vi "Read Inputs from system.vi"(8 "error in":errorcluster, 11 "GPIC Core runtime in":refnum<class "GPIC Core runtime.lvclass">) -> (0 "error out":errorcluster, 2 "Inputs from system":T1, 3 "GPIC Core runtime out":refnum<class "GPIC Core runtime.lvclass">)   [LabVIEW 2017, in "GPIC Core runtime.lvclass"]
uses:
  GPIC Core runtime.lvclass
  configuration/input data indices.ctl
  GPIC Core runtime.lvclass/GPIC Core runtime.ctl
  configuration/GPIC Core configuration.lvclass
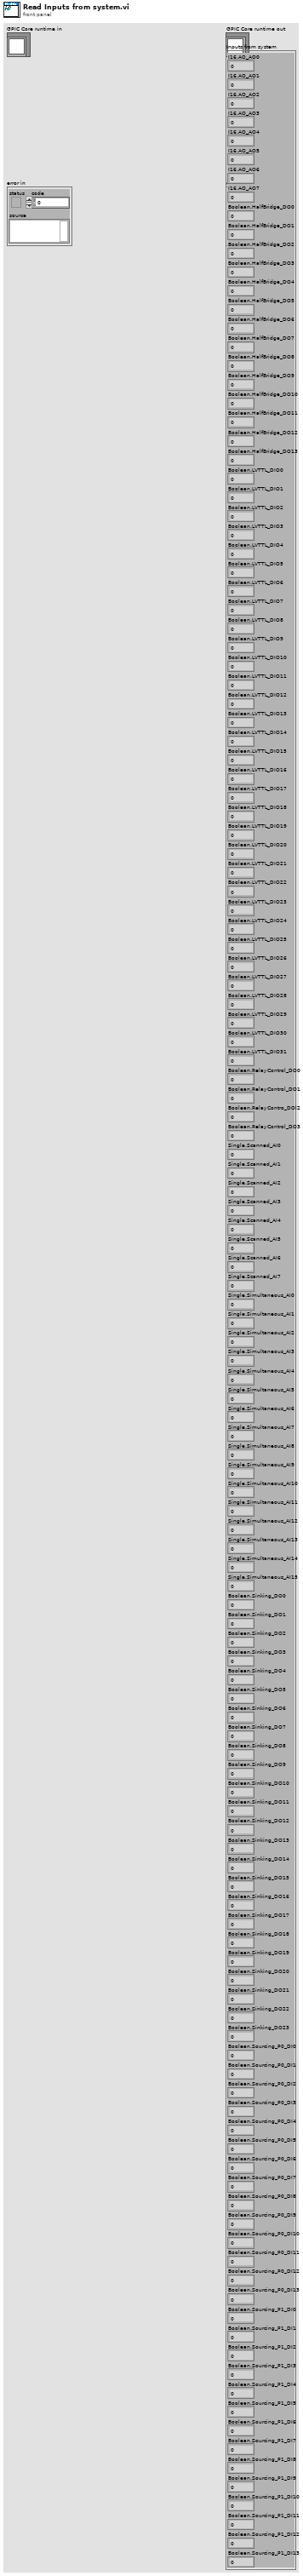
[diagram p1: front panel]
types:
  T1 = typedef "GPIC Core configuration.lvclass/input data indices.ctl" = cluster{"I16.AO_AO0":i32, "I16.AO_AO1":i32, "I16.AO_AO2":i32, "I16.AO_AO3":i32, "I16.AO_AO4":i32, "I16.AO_AO5":i32, "I16.AO_AO6":i32, "I16.AO_AO7":i32, "Boolean.HalfBridge_DO0":i32, "Boolean.HalfBridge_DO1":i32, "Boolean.HalfBridge_DO2":i32, "Boolean.HalfBridge_DO3":i32, "Boolean.HalfBridge_DO4":i32, "Boolean.HalfBridge_DO5":i32, "Boolean.HalfBridge_DO6":i32, "Boolean.HalfBridge_DO7":i32, "Boolean.HalfBridge_DO8":i32, "Boolean.HalfBridge_DO9":i32, "Boolean.HalfBridge_DO10":i32, "Boolean.HalfBridge_DO11":i32, "Boolean.HalfBridge_DO12":i32, "Boolean.HalfBridge_DO13":i32, "Boolean.LVTTL_DIO0":i32, "Boolean.LVTTL_DIO1":i32, "Boolean.LVTTL_DIO2":i32, "Boolean.LVTTL_DIO3":i32, "Boolean.LVTTL_DIO4":i32, "Boolean.LVTTL_DIO5":i32, "Boolean.LVTTL_DIO6":i32, "Boolean.LVTTL_DIO7":i32, "Boolean.LVTTL_DIO8":i32, "Boolean.LVTTL_DIO9":i32, "Boolean.LVTTL_DIO10":i32, "Boolean.LVTTL_DIO11":i32, "Boolean.LVTTL_DIO12":i32, "Boolean.LVTTL_DIO13":i32, "Boolean.LVTTL_DIO14":i32, "Boolean.LVTTL_DIO15":i32, "Boolean.LVTTL_DIO16":i32, "Boolean.LVTTL_DIO17":i32, "Boolean.LVTTL_DIO18":i32, "Boolean.LVTTL_DIO19":i32, "Boolean.LVTTL_DIO20":i32, "Boolean.LVTTL_DIO21":i32, "Boolean.LVTTL_DIO22":i32, "Boolean.LVTTL_DIO23":i32, "Boolean.LVTTL_DIO24":i32, "Boolean.LVTTL_DIO25":i32, "Boolean.LVTTL_DIO26":i32, "Boolean.LVTTL_DIO27":i32, "Boolean.LVTTL_DIO28":i32, "Boolean.LVTTL_DIO29":i32, "Boolean.LVTTL_DIO30":i32, "Boolean.LVTTL_DIO31":i32, "Boolean.RelayControl_DO0":i32, "Boolean.RelayControl_DO1":i32, "Boolean.RelayContro_DOl2":i32, "Boolean.RelayControl_DO3":i32, "Single.Scanned_AI0":i32, "Single.Scanned_AI1":i32, "Single.Scanned_AI2":i32, "Single.Scanned_AI3":i32, "Single.Scanned_AI4":i32, "Single.Scanned_AI5":i32, "Single.Scanned_AI6":i32, "Single.Scanned_AI7":i32, "Single.Simultaneous_AI0":i32, "Single.Simultaneous_AI1":i32, "Single.Simultaneous_AI2":i32, "Single.Simultaneous_AI3":i32, "Single.Simultaneous_AI4":i32, "Single.Simultaneous_AI5":i32, "Single.Simultaneous_AI6":i32, "Single.Simultaneous_AI7":i32, "Single.Simultaneous_AI8":i32, "Single.Simultaneous_AI9":i32, "Single.Simultaneous_AI10":i32, "Single.Simultaneous_AI11":i32, "Single.Simultaneous_AI12":i32, "Single.Simultaneous_AI13":i32, "Single.Simultaneous_AI14":i32, "Single.Simultaneous_AI15":i32, "Boolean.Sinking_DO0":i32, "Boolean.Sinking_DO1":i32, "Boolean.Sinking_DO2":i32, "Boolean.Sinking_DO3":i32, "Boolean.Sinking_DO4":i32, "Boolean.Sinking_DO5":i32, "Boolean.Sinking_DO6":i32, "Boolean.Sinking_DO7":i32, "Boolean.Sinking_DO8":i32, "Boolean.Sinking_DO9":i32, "Boolean.Sinking_DO10":i32, "Boolean.Sinking_DO11":i32, "Boolean.Sinking_DO12":i32, "Boolean.Sinking_DO13":i32, "Boolean.Sinking_DO14":i32, "Boolean.Sinking_DO15":i32, "Boolean.Sinking_DO16":i32, "Boolean.Sinking_DO17":i32, "Boolean.Sinking_DO18":i32, "Boolean.Sinking_DO19":i32, "Boolean.Sinking_DO20":i32, "Boolean.Sinking_DO21":i32, "Boolean.Sinking_DO22":i32, "Boolean.Sinking_DO23":i32, "Boolean.Sourcing_P0_DI0":i32, "Boolean.Sourcing_P0_DI1":i32, "Boolean.Sourcing_P0_DI2":i32, "Boolean.Sourcing_P0_DI3":i32, "Boolean.Sourcing_P0_DI4":i32, "Boolean.Sourcing_P0_DI5":i32, "Boolean.Sourcing_P0_DI6":i32, "Boolean.Sourcing_P0_DI7":i32, "Boolean.Sourcing_P0_DI8":i32, "Boolean.Sourcing_P0_DI9":i32, "Boolean.Sourcing_P0_DI10":i32, "Boolean.Sourcing_P0_DI11":i32, "Boolean.Sourcing_P0_DI12":i32, "Boolean.Sourcing_P0_DI13":i32, "Boolean.Sourcing_P1_DI0":i32, "Boolean.Sourcing_P1_DI1":i32, "Boolean.Sourcing_P1_DI2":i32, "Boolean.Sourcing_P1_DI3":i32, "Boolean.Sourcing_P1_DI4":i32, "Boolean.Sourcing_P1_DI5":i32, "Boolean.Sourcing_P1_DI6":i32, "Boolean.Sourcing_P1_DI7":i32, "Boolean.Sourcing_P1_DI8":i32, "Boolean.Sourcing_P1_DI9":i32, "Boolean.Sourcing_P1_DI10":i32, "Boolean.Sourcing_P1_DI11":i32, "Boolean.Sourcing_P1_DI12":i32, "Boolean.Sourcing_P1_DI13":i32}
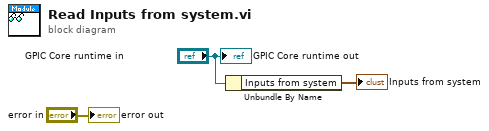
[diagram p0: block diagram]
diagram:
  n1 = Unbundle By Name("GPIC Core runtime in") -> ("Inputs from system"=→"Inputs from system":T1)
  "error out" <- "error in"
  "GPIC Core runtime out" <- "GPIC Core runtime in"
